vi "Handle Message.vi"(5 "Stack ID":u8, 7 "Function ID":u8, 8 "error in (no error)":errorcluster, 10 "Data":string, 11 "Humidity Bricklet in":refnum<class "Humidity Bricklet.lvclass">) -> (0 "error out":errorcluster, 1 "Send Answer":bool, 2 "Answer":variant, 3 "Humidity Bricklet out":refnum<class "Humidity Bricklet.lvclass">)   [LabVIEW 2011, in "Tinkerforge.lvlib" / "Humidity Bricklet.lvclass"]
doc: "This VI is the child implementation of \"Handle Message.vi\" and processes all responses for this device type."
uses:
  Humidity Bricklet.lvclass
  Humidity Bricklet.lvclass/Humidity Bricklet.ctl
  Device/Device.lvclass
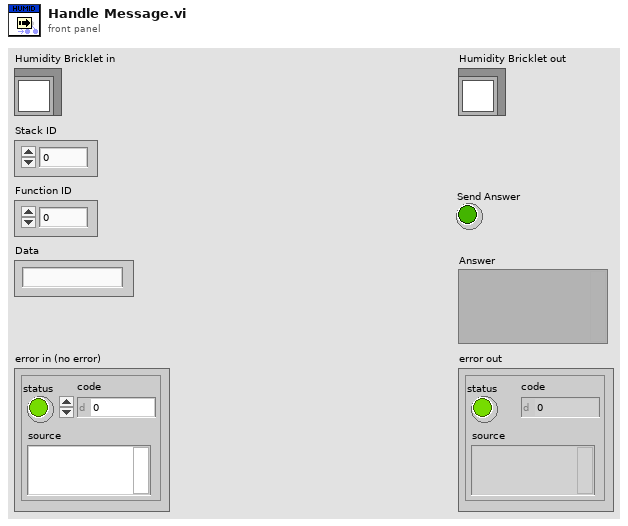
[diagram p1: front panel]
types:
  T1 = typedef "Tinkerforge.lvlib/Device.lvclass/Callback Threshold.ctl" = cluster{"Callback Option":T2, "min":i16, "max":i16}
  T2 = typedef "Tinkerforge.lvlib/Device.lvclass/Callback Option.ctl" = enum8{"CB off", "outside range", "inside range", "smaller", "greater"}
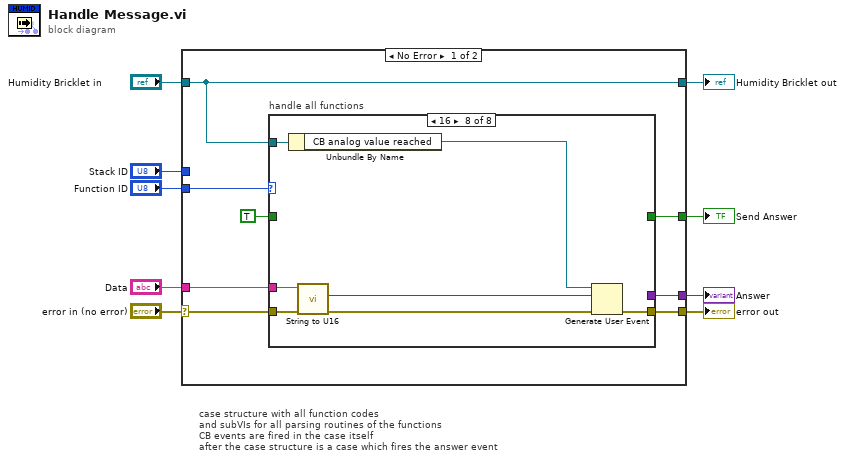
[diagram p0: block diagram]
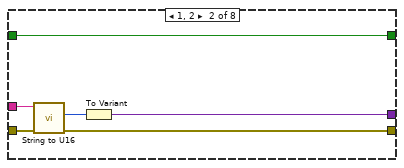
[diagram p3: hidden frame]
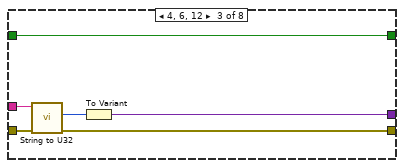
[diagram p4: hidden frame]
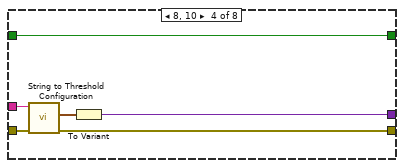
[diagram p5: hidden frame]
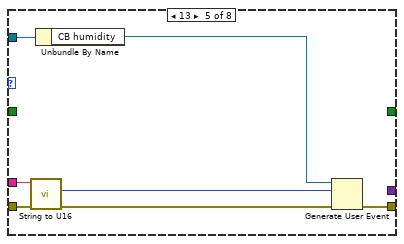
[diagram p6: hidden frame]
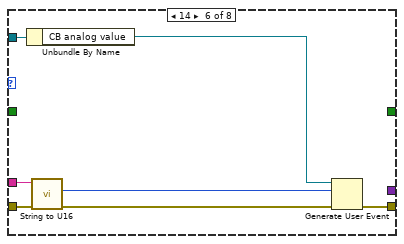
[diagram p7: hidden frame]
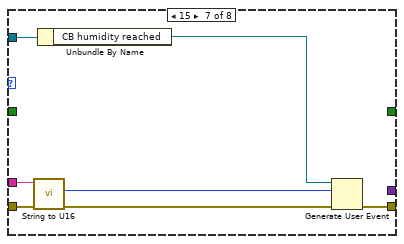
[diagram p8: hidden frame]
diagram:
  # "case structure with all function codes\nand subVIs for all parsing routines of the functions\nCB events are fired in the case itself\nafter the case structure is a case which fires the answer event"
  n1 = case shown="No Error" "error in (no error)" {
    selector: "error in (no error)" -> [w13 w64]
    tunnel: "Humidity Bricklet in" -> [w17 w65]
    tunnel: "Stack ID" -> [_ _]
    tunnel: "Function ID" -> [w16 _]
    tunnel: "Data" -> [w14 _]
    tunnel: [w17 w65] -> w4
    tunnel: [w11 w64] -> w3
    tunnel: [w12 _] -> w2
    tunnel: [w10 _] -> w1
    frame No Error {
      n2 = case "handle all functions" shown="16" w16 {
        tunnel: w13 -> [_ w21 w27 w33 w39 w46 w53 w60]
        tunnel: w14 -> [_ w20 w26 w31 w38 w45 w52 w59]
        tunnel: TRUE -> [_ w23 w29 w35 _ _ _ _]
        tunnel: [_ w23 w29 w35 _ _ _ _] -> w10
        tunnel: [_ w19 w25 w32 w40 w47 w54 w61] -> w11
        tunnel: [_ w22 w28 w34 _ _ _ _] -> w12
        tunnel: w17 -> [_ _ _ _ w42 w49 w56 w63]
        frame Default {
          # "nothing to do"
        }
        frame 1, 2 {
          n3 = call "String to U16.vi"("Error In"=w21, "String"=w20) -> ("Error Out"=w19:errorcluster, "U16"=w18:u16)  [unwired: 7 in, 1 out]
          n4 = To Variant(anything=w18) -> (Variant=w22:variant)
        }
        frame 4, 6, 12 {
          n5 = call "String to U32.vi"("Error In"=w27, "String"=w26) -> ("Error Out"=w25:errorcluster, "U32"=w24:u32)  [unwired: 7 in, 1 out]
          n6 = To Variant(anything=w24) -> (Variant=w28:variant)
        }
        frame 8, 10 {
          n7 = call "String to Threshold Configuration.vi"("Error In"=w33, "String"=w31) -> ("Error Out"=w32:errorcluster, "Callback Threshold"=w30:T1)  [unwired: 7 in, 1 out]
          n8 = To Variant(anything=w30) -> (Variant=w34:variant)
        }
        frame 13 {
          n9 = call "String to U16.vi"("Error In"=w39, "String"=w38) -> ("Error Out"=w37:errorcluster, "U16"=w36:u16)  [unwired: 7 in, 1 out]
          n10 = Unbundle By Name(w42) -> ("CB humidity"=w41:refnum<user-event>)
          n11 = Generate User Event(user event=w41, event data cluster=w36, error in=w37) -> (error out=w40:errorcluster)  [unwired: 1 out]
        }
        frame 14 {
          n12 = Unbundle By Name(w49) -> ("CB analog value"=w48:refnum<user-event>)
          n13 = call "String to U16.vi"("Error In"=w46, "String"=w45) -> ("Error Out"=w43:errorcluster, "U16"=w44:u16)  [unwired: 7 in, 1 out]
          n14 = Generate User Event(user event=w48, event data cluster=w44, error in=w43) -> (error out=w47:errorcluster)  [unwired: 1 out]
        }
        frame 15 {
          n15 = call "String to U16.vi"("Error In"=w53, "String"=w52) -> ("Error Out"=w50:errorcluster, "U16"=w51:u16)  [unwired: 7 in, 1 out]
          n16 = Unbundle By Name(w56) -> ("CB humidity reached"=w55:refnum<user-event>)
          n17 = Generate User Event(user event=w55, event data cluster=w51, error in=w50) -> (error out=w54:errorcluster)  [unwired: 1 out]
        }
        frame 16 {
          n18 = Unbundle By Name(w63) -> ("CB analog value reached"=w62:refnum<user-event>)
          n19 = call "String to U16.vi"("Error In"=w60, "String"=w59) -> ("Error Out"=w58:errorcluster, "U16"=w57:u16)  [unwired: 7 in, 1 out]
          n20 = Generate User Event(user event=w62, event data cluster=w57, error in=w58) -> (error out=w61:errorcluster)  [unwired: 1 out]
        }
      }
    }
    frame Error {
    }
  }
  "error out" <- w3
  "Humidity Bricklet out" <- w4
  "Answer" <- w2
  "Send Answer" <- w1
